vi "GlobalVariables.vi"() -> ()   [LabVIEW 2013]
panel:
  out "Wall Position Reset Global":bool
  in  "Wall Position Global":dbl
  in  "Recording Folder":path
  in  "SessionID":string
  in  "save data":bool
  in  "prepare recording":bool
  in  "quit program":bool
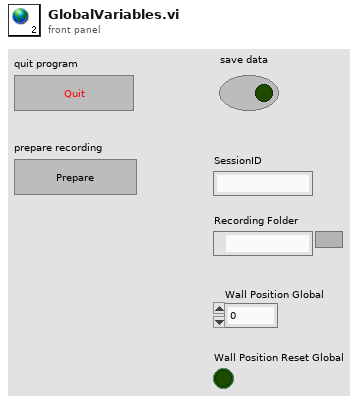
[diagram p1: front panel]
diagram:
